vi "FrontPanelManager_CleanUp.vi"(5 "error in (no error)":errorcluster) -> (19 "error out":errorcluster)   [LabVIEW 2014, in "FrontPanelManager.lvclass"]
uses:
  FrontPanelManager.lvclass
  WebFrontPanel_class/WebFrontPanel.lvclass
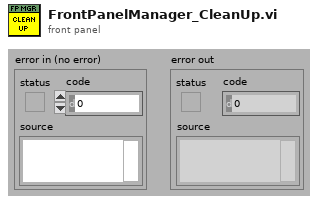
[diagram p1: front panel]
types:
  T1 = typedef "FrontPanelManager.lvclass/ObjectAttributes.ctl" = cluster{"WebFrontPanels":refnum<class "WebFrontPanel.lvclass">[], "WFP Names":string[], "Root folder":path}
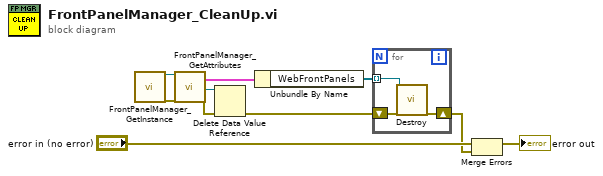
[diagram p0: block diagram]
diagram:
  n1 = call "FrontPanelManager_GetInstance.vi"() -> ("reference out"=w7:refnum<class "FrontPanelManager.lvclass">, "error out"=w8:errorcluster)  [unwired: 15 in, 3 out]
  n2 = call "FrontPanelManager_GetAttributes.vi"("reference in"=w7, "error in (no error)"=w8) -> ("Data"=w3:T1, "DataRef"=w5:refnum<data-value>, "error out"=w6:errorcluster)  [unwired: 14 in, 1 out]
  n3 = Delete Data Value Reference(data value reference=w5, error in=w6) -> (error out=w1:errorcluster)  [unwired: 1 out]
  n4 = Unbundle By Name(w3) -> ("WebFrontPanels"=w2:refnum<class "WebFrontPanel.lvclass">[])
  n5 = for {
    tunnel: w2 -> [w12] mode=indexing
    shift-right: [w10] -> _
    shift-left: w1 -> [w11]
    n6 = call-dynamic "Destroy.vi"("reference in"=w12, "error in (no error)"=w11) -> ("error out"=w10:errorcluster)  [unwired: 16 in, 1 out]
  }
  n7 = Merge Errors("error in (no error)", w1) -> (→"error out":errorcluster)
